vi "SetM2PositionPID.vi"(0 "VISA Refnum in":refnum<visa-resource-name>, 1 "Kd":u32 max=127 step=1, 2 "KiMax":u32 max=127 step=1, 3 "Deadzone":u32 max=127 step=1, 5 "Ki":u32 max=127 step=1, 7 "Kp":u32 max=127 step=1, 9 "Address":u8, 11 "error in (no error)":errorcluster, 12 "MaxPos":i32 max=127 step=1, 13 "MinPos":i32 max=127 step=1) -> (4 "VISA Refnum out":refnum<visa-resource-name>, 6 "Valid":bool, 15 "error out":errorcluster)   [LabVIEW 2015, in "Ion Motion Roboclaw.lvlib"]
uses:
  <instrlib>/Ion Motion Roboclaw/Ion Motion Roboclaw.lvlib
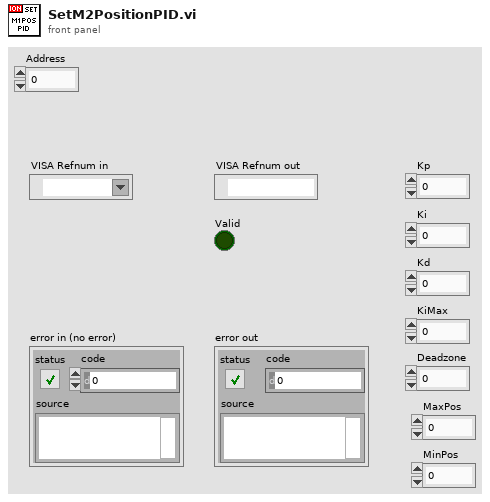
[diagram p1: front panel]
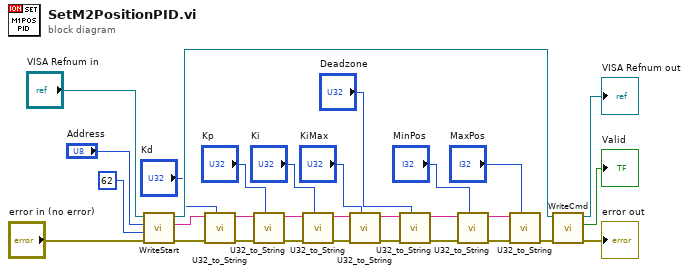
[diagram p0: block diagram]
diagram:
  n1 = call <instrlib>:"WriteStart.vi"("error in (no error)"="error in (no error)", "Cmd"=u8 62, "Address"="Address", "VISA Refnum in"="VISA Refnum in") -> ("error out"=w18:errorcluster, "String Out"=w16:string, "VISA Refnum out"=w29:refnum<visa-resource-name>)  [unwired: 5 in]
  n2 = call <instrlib>:"U32_to_String.vi"("number"="Kd", "error in (no error)"=w18, "String In"=w16) -> ("error out"=w19:errorcluster, "String Out"=w15:string)  [unwired: 5 in]
  n3 = call <instrlib>:"U32_to_String.vi"("number"="Kp", "error in (no error)"=w19, "String In"=w15) -> ("error out"=w20:errorcluster, "String Out"=w14:string)  [unwired: 5 in]
  n4 = call <instrlib>:"U32_to_String.vi"("number"="Ki", "error in (no error)"=w20, "String In"=w14) -> ("error out"=w21:errorcluster, "String Out"=w13:string)  [unwired: 5 in]
  n5 = call <instrlib>:"U32_to_String.vi"("number"="KiMax", "error in (no error)"=w21, "String In"=w13) -> ("error out"=w22:errorcluster, "String Out"=w12:string)  [unwired: 5 in]
  n6 = call <instrlib>:"U32_to_String.vi"("number"="Deadzone", "error in (no error)"=w22, "String In"=w12) -> ("error out"=w23:errorcluster, "String Out"=w11:string)  [unwired: 5 in]
  n7 = call <instrlib>:"U32_to_String.vi"("number"="MinPos", "error in (no error)"=w23, "String In"=w11) -> ("error out"=w24:errorcluster, "String Out"=w10:string)  [unwired: 5 in]
  n8 = call <instrlib>:"U32_to_String.vi"("number"="MaxPos", "error in (no error)"=w24, "String In"=w10) -> ("error out"=w25:errorcluster)  [unwired: 5 in, 1 out]
  n9 = call <instrlib>:"WriteCmd.vi"("error in (no error)"=w25, "VISA Refnum in"=w29) -> ("error out"=→"error out":errorcluster, "Valid"=→"Valid":bool, "VISA Refnum out"=→"VISA Refnum out":refnum<visa-resource-name>)  [unwired: 3 in]
